vi "Configure Digital SSI Output.vi"(8 "error in (no error)":errorcluster, 9 "SSI Output Sync Delay (0 us)":dbl, 10 "SSI Output Bits Per Frame (32)":i32=32, 11 "VISA resource name":refnum<visa-resource-name>) -> (0 "error out":errorcluster, 3 "VISA resource name out":refnum<visa-resource-name>)   [LabVIEW 2018, in "Agilent PSG MXG Series.lvlib"]
doc: "Configures SSI output.\n\n\n<b>Note:</b>\nIt is only valid in N5172B/82B with <b>Option 003</b> or <b>Option 004</b> or <b>Option both</b>."
uses:
  Agilent PSG MXG Series.lvlib
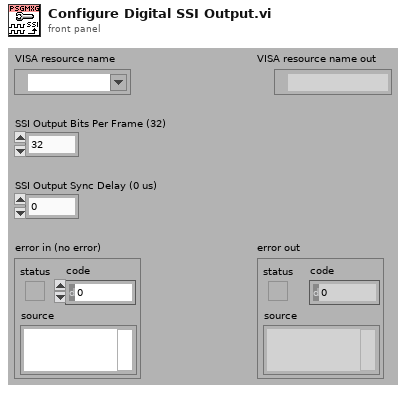
[diagram p1: front panel]
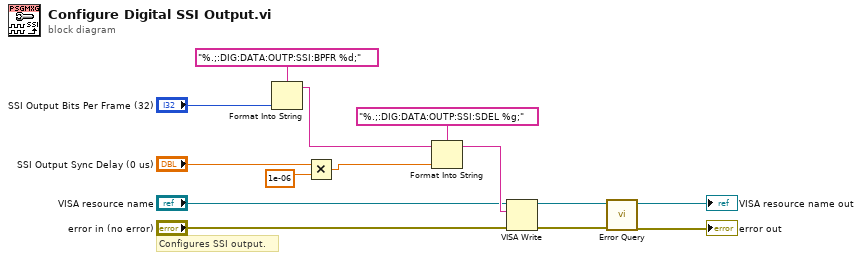
[diagram p0: block diagram]
diagram:
  # "Configures SSI output."
  n1 = Format Into String(format string="%.;:DIG:DATA:OUTP:SSI:BPFR %d;", "SSI Output Bits Per Frame (32)") -> (resulting string=w12:string)  [unwired: 2 in, 1 out]
  n2 = Multiply(x="SSI Output Sync Delay (0 us)", y=1e-06) -> (x*y=w1:dbl)
  n3 = Format Into String(format string="%.;:DIG:DATA:OUTP:SSI:SDEL %g;", initial string=w12, w1) -> (resulting string=w10:string)  [unwired: 1 in, 1 out]
  n4 = VISA Write(VISA resource name="VISA resource name", write buffer=w10, error in (no error)="error in (no error)") -> (VISA resource name out=w7:refnum<visa-resource-name>, error out=w6:errorcluster)  [unwired: 1 out]
  n5 = call "Error Query.vi"("error in (no error)"=w6, "VISA resource name"=w7) -> ("error out"=→"error out":errorcluster, "VISA resource name out"=→"VISA resource name out":refnum<visa-resource-name>)  [unwired: 6 in, 2 out]
